vi "Retrieve Data from Device.vi"(8 "error in (no error)":errorcluster, 11 "Aperiodic DAQ in":refnum<class "Aperiodic DAQ.lvclass">=refnum) -> (0 "error out":errorcluster, 2 "Data":refnum<class "Data.lvclass">, 3 "Aperiodic DAQ out":refnum<class "Aperiodic DAQ.lvclass">)   [LabVIEW 2014, in "Aperiodic DAQ.lvclass"]
uses:
  Aperiodic DAQ.lvclass
  Data/Data.lvclass
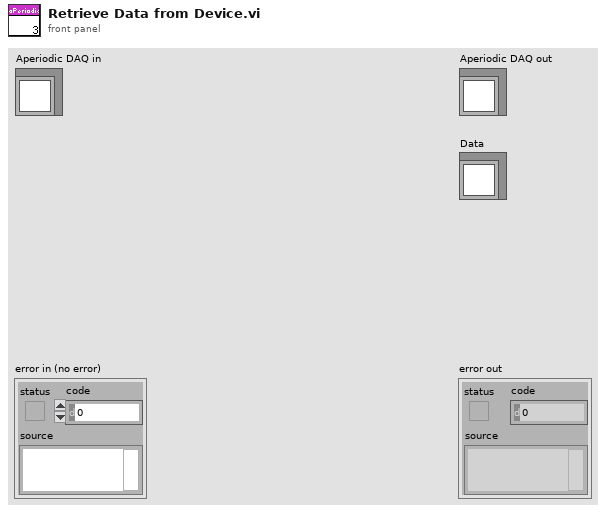
[diagram p1: front panel]
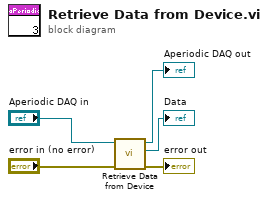
[diagram p0: block diagram]
diagram:
  n1 = call-parent "Retrieve Data from Device.vi"("error in (no error)"="error in (no error)", "DAQ Device in"="Aperiodic DAQ in") -> ("error out"=→"error out":errorcluster, "Data"=→"Data":refnum<class "Data.lvclass">, "DAQ Device out"=→"Aperiodic DAQ out":refnum<class "Aperiodic DAQ.lvclass">)  [unwired: 7 in]
